vi "continuousSamplingFPGA.vi"() -> ()   [LabVIEW 2012]
uses:
  <vilib>/rvi/Emulation/niFpgaSctlEmulationGetInTimedLoop.vi
  <vilib>/rvi/Emulation/niFpgaSctlEmulationGlobalWrite.vi
  <vilib>/rvi/interface/RandomDataEmulation/nirviRandomDataFPGAFIFO.vi
  <vilib>/rvi/interface/RandomDataEmulation/niFpgaRandomDataHandleErrors.vi
  <vilib>/rvi/eio/common/nirviEmuTemplateMethod_errors.vi
  <vilib>/rvi/DataTransferAndStorage/Container/XNode/niFpgaContainer.xnode
  <vilib>/rvi/interface/RandomDataEmulation/nirviRandomDataFpgaReadWriteTemplate.vi
  <vilib>/eio/EIONode/EIONode.xnode
panel:
  out "z target":bool
  in  "deflection threshold":fxp<+/-,64,32>
  in  "z threshold":fxp<+/-,64,32>
  out "xy target":bool
  in  "y threshold":fxp<+,32,17>
  in  "x threshold":fxp<+,32,17>
  out "z sensor":fxp<+/-,20,5>
  in  "z control":T1
  in  "dataRefresh Clock (uSec)":fxp<+/-,64,29>
  out "Timed Out?":bool
  out "direction":u16
  in  "XY Clock (uSec)":fxp<+/-,64,29>
  out "y sensor":fxp<+/-,20,5>
  out "y output":fxp<+/-,64,29>
  in  "y control":T1
  out "x sensor":fxp<+/-,20,5>
  out "x output":fxp<+/-,64,29>
  in  "x control":T1
  out "deflection sensor":fxp<+/-,20,5>
  out "z output":fxp<+/-,64,29>
  in  "deflection control":T1
  in  "Z Clock (uSec)":fxp<+/-,64,29>
  out "length":u16
  out "y_pos":u16
  out "x_pos":u16
  out "ToRead":u32
  out "signalToStop":bool
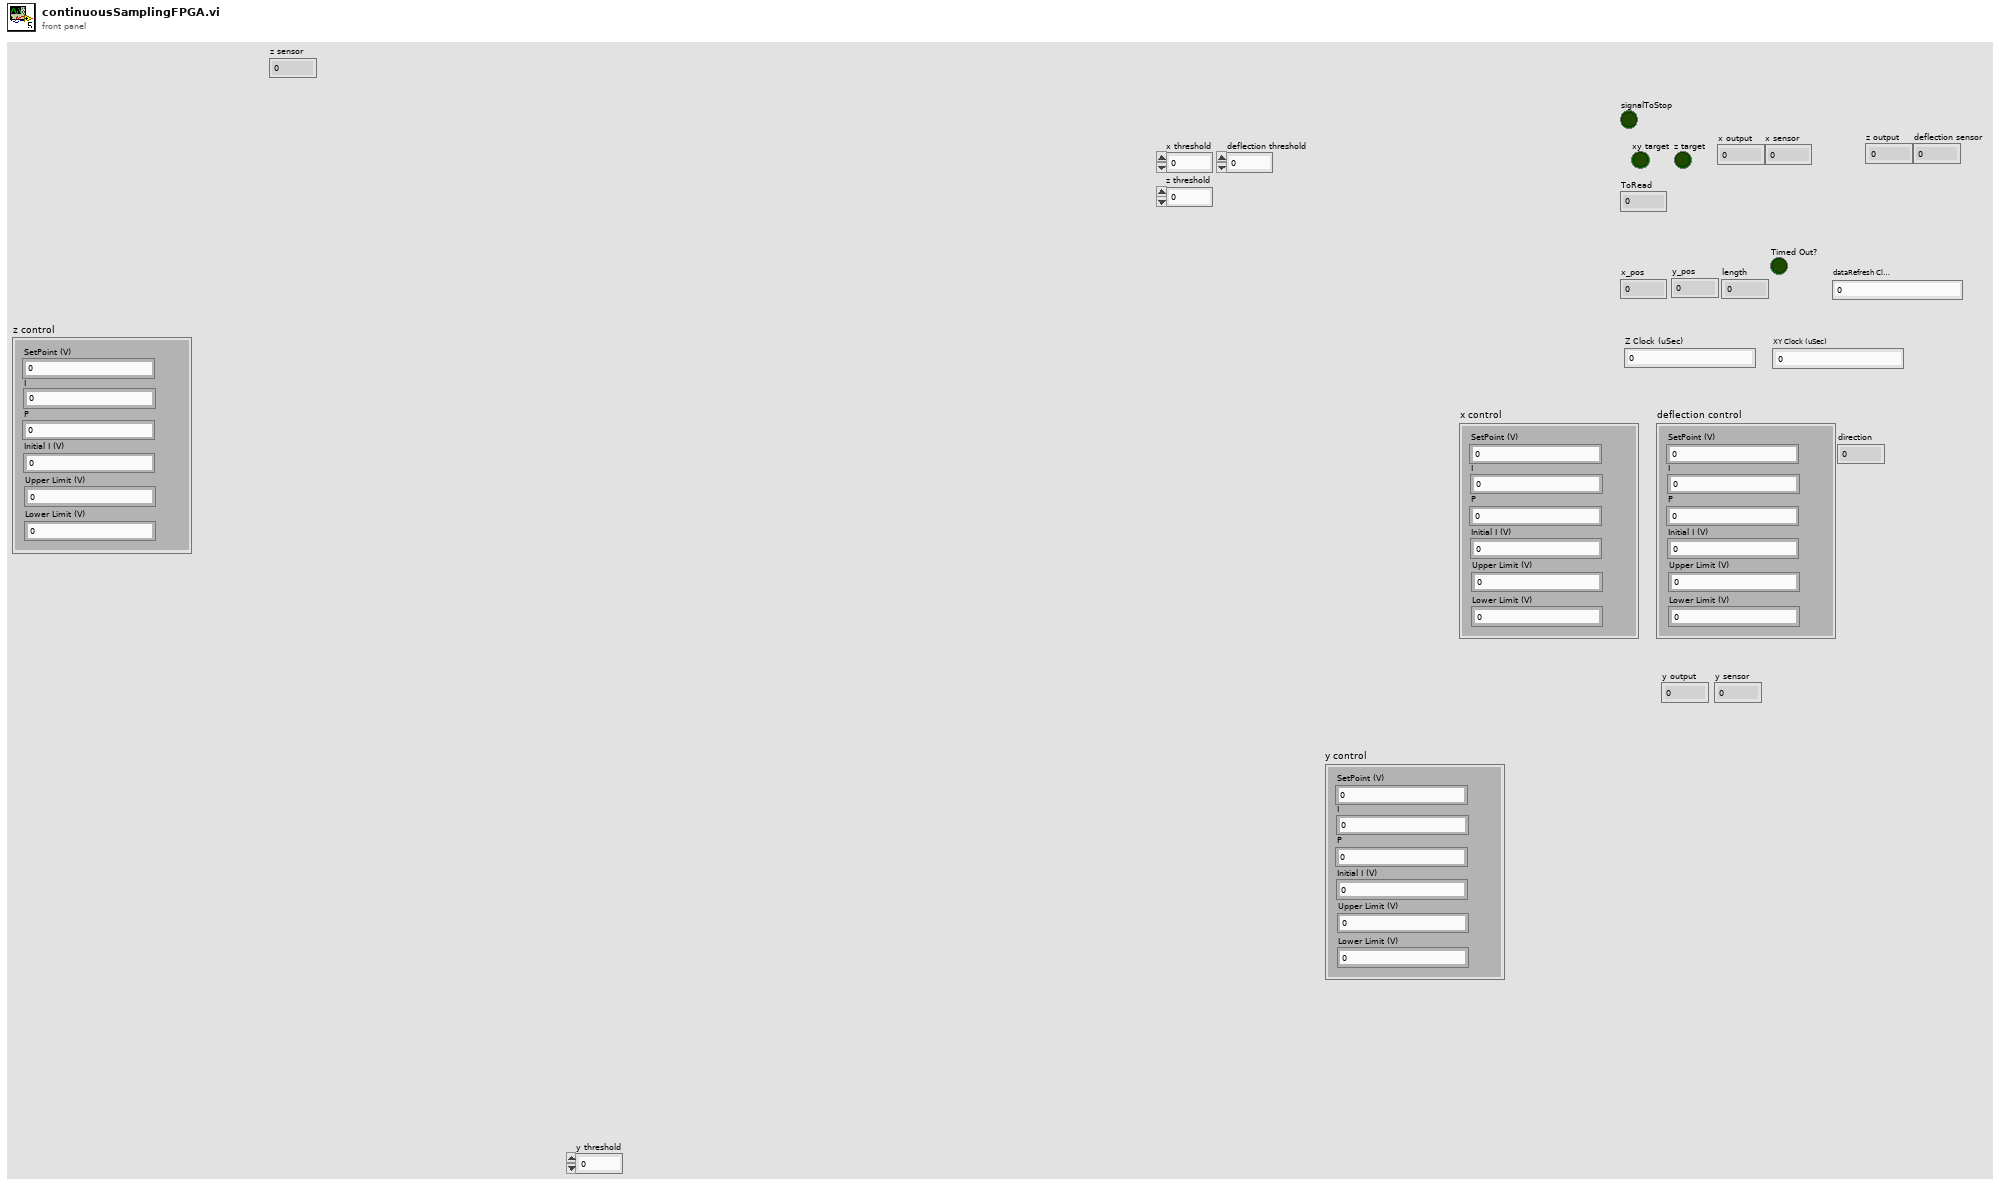
[diagram p1: front panel]
types:
  T1 = cluster{"SetPoint (V)":fxp<+/-,20,5>, "I":fxp<+/-,20,5>, "P":fxp<+/-,20,5>, "Initial I (V)":fxp<+/-,64,29>, "Upper Limit (V)":fxp<+/-,64,29>, "Lower Limit (V)":fxp<+/-,64,29>}
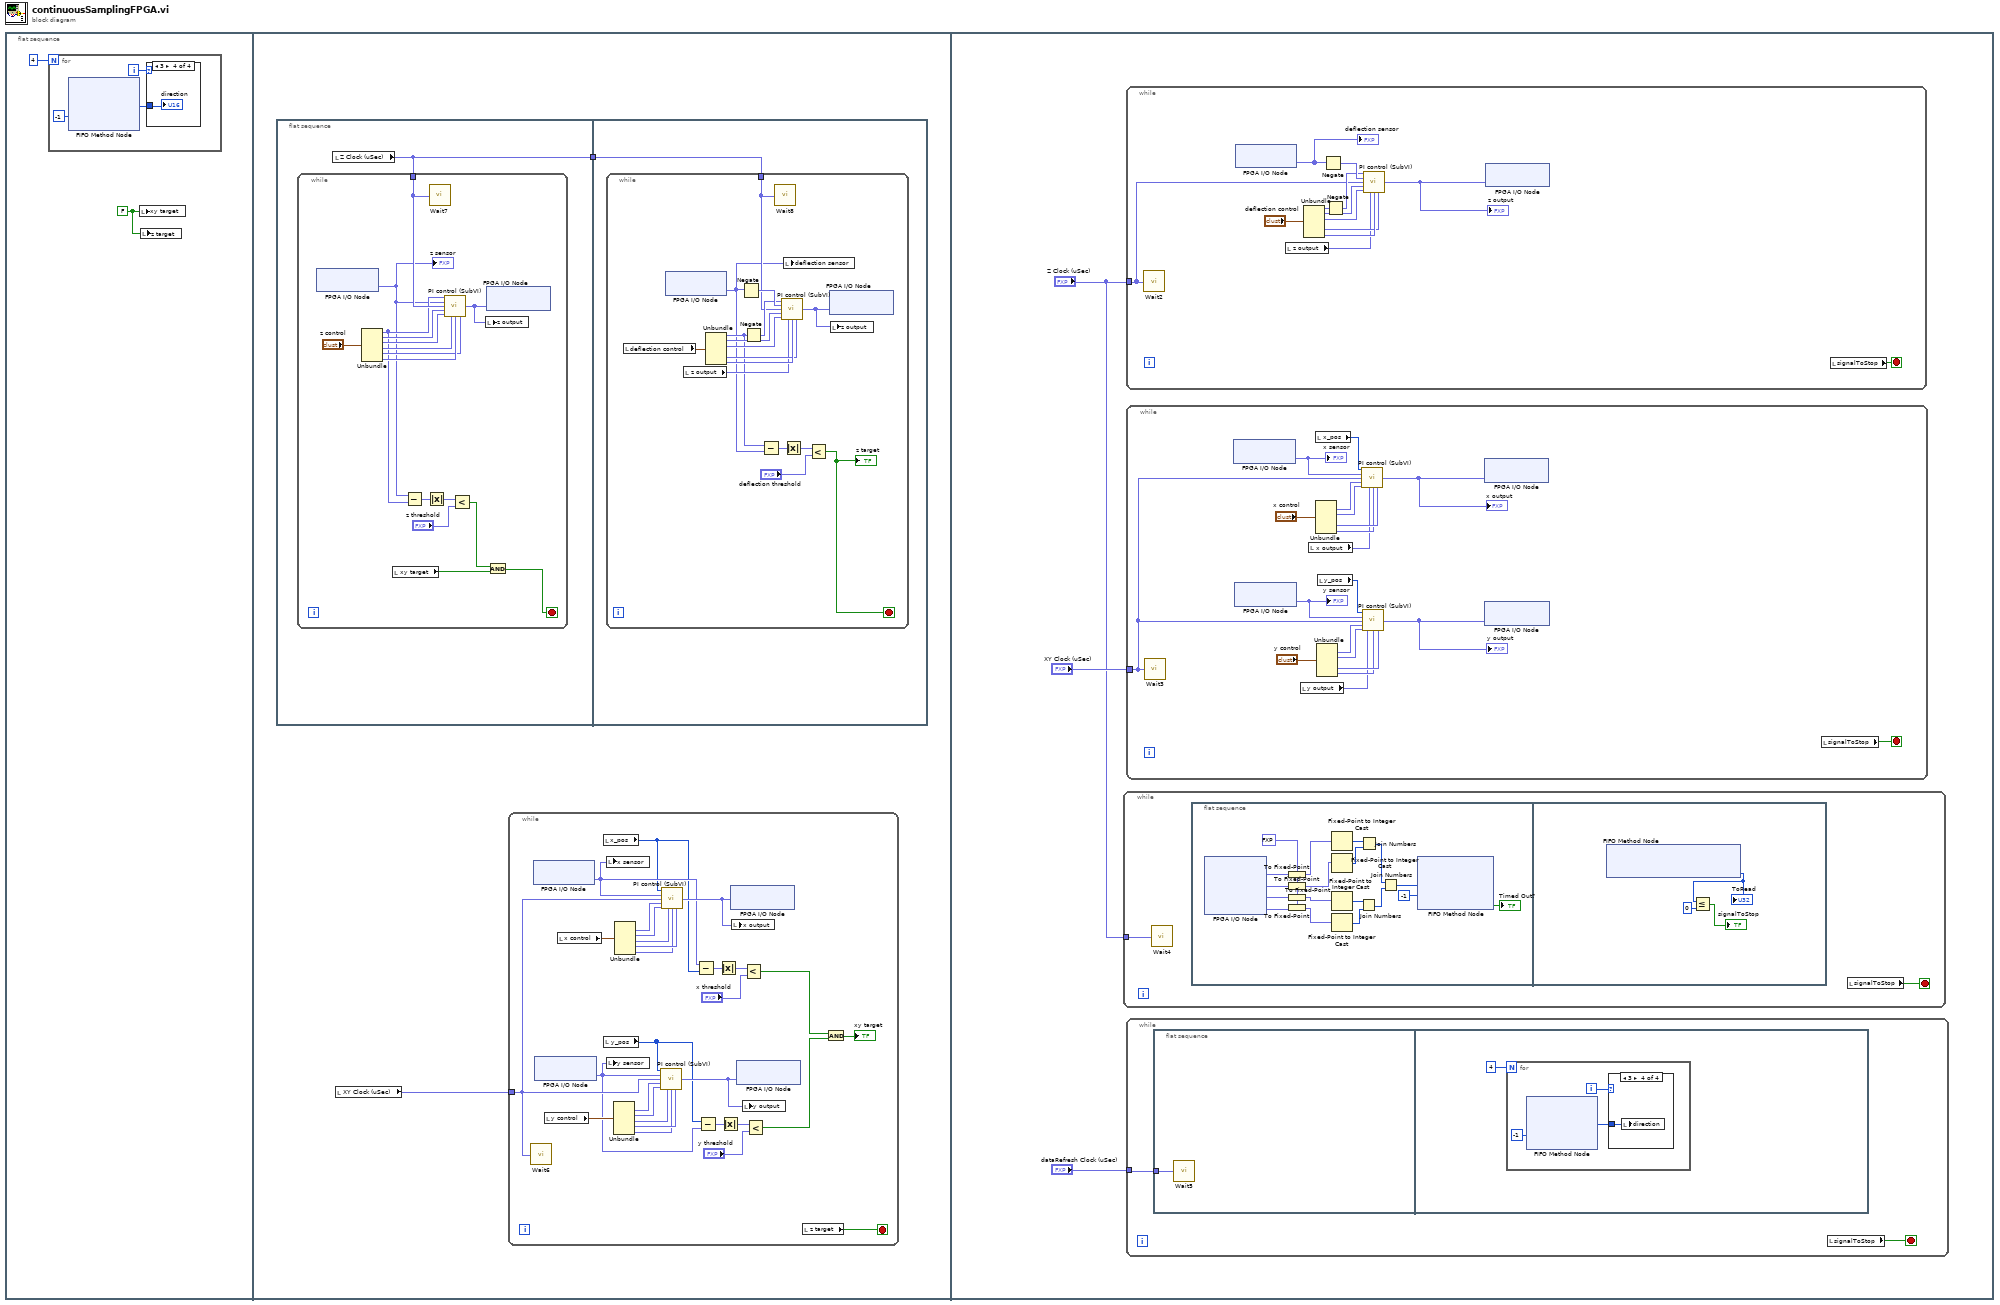
[diagram p0: block diagram]
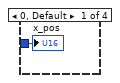
[diagram p2: hidden frame]
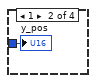
[diagram p3: hidden frame]
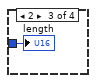
[diagram p4: hidden frame]
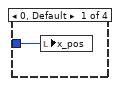
[diagram p5: hidden frame]
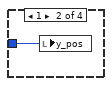
[diagram p6: hidden frame]
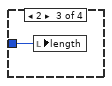
[diagram p7: hidden frame]
diagram:
  n1 = flat-sequence {
    frame #0 {
      w1 = FALSE ("xy target")
      n2 = for {
        N: 4 -> [_]
        i -> [w5]
        n3 = xnode ("FIFO Method Node")("Timeout"=-1) -> ("Element"=w3:u16)  [unwired: 1 in, 2 out]
        n4 = case shown="3" w5 {
          tunnel: w3 -> [w6 w7 w8 w9]
          frame 0, Default {
            "x_pos" <- w6
          }
          frame 1 {
            "y_pos" <- w7
          }
          frame 2 {
            "length" <- w8
          }
          frame 3 {
            "direction" <- w9
          }
        }
      }
      n5 = local write "xy target"(w1) -> ()
      n6 = local write "z target"(w1) -> ()
    }
    frame #1 {
      n7 = flat-sequence {
        tunnel: [w12] -> w10
        tunnel: w10 -> [w29]
        frame #0 {
          n8 = local read "Z Clock (uSec)"() -> (w12:fxp<+/-,64,29>)
          n9 = while {
            tunnel: w12 -> [w21]
            stop <- w19 stop-if-true
            n10 = xnode "FPGA I/O Node"() -> ("Mod1/AI2"=w14:fxp<+/-,20,5>)  [unwired: 1 in, 1 out]
            "z sensor" <- w14
            n11 = Unbundle("z control") -> ("SetPoint (V)"=w15:fxp<+/-,20,5>, "I"=w28:fxp<+/-,20,5>, "P"=w27:fxp<+/-,20,5>, "Initial I (V)"=w26:fxp<+/-,64,29>, "Upper Limit (V)"=w24:fxp<+/-,64,29>, "Lower Limit (V)"=w25:fxp<+/-,64,29>)
            n12 = local read "xy target"() -> (w20:bool)
            n13 = Subtract(x=w14, y=w15) -> (x-y=w18:fxp<+/-,21,6>)
            n14 = Absolute Value(x=w18) -> (abs(x)=w17:fxp<+,20,5>)
            n15 = call "Wait7"("Count(uSec)"=w21) -> ()  [unwired: 1 out]
            n16 = call "PI control (SubVI).vi"("SetPoint"=w15, "Feedback"=w14, "Clock"=w21, "I"=w28, "P"=w27, "Initial I"=w26, "Lower Limit"=w25, "Upper Limit in"=w24) -> ("Output"=w22:fxp<+/-,64,29>)  [unwired: 7 in]
            n17 = Less?(x=w17, y="z threshold") -> (x < y?=w13:bool)
            n18 = local write "z output"(w22) -> ()
            n19 = xnode "FPGA I/O Node"("Mod8/AO2"=w22) -> ()  [unwired: 1 in, 1 out]
            n20 = And(x=w13, y=w20) -> (x .and. y?=w19:bool)
          }
        }
        frame #1 {
          n21 = while {
            tunnel: w29 -> [w37]
            stop <- w30 stop-if-true
            n22 = local read "deflection control"() -> (w38:T1)
            n23 = xnode "FPGA I/O Node"() -> ("Mod1/AI3"=w31:fxp<+/-,20,5>)  [unwired: 1 in, 1 out]
            n24 = local read "z output"() -> (w36:fxp<+/-,64,29>)
            n25 = Unbundle(w38) -> ("SetPoint (V)"=w32:fxp<+/-,20,5>, "I"=w45:fxp<+/-,20,5>, "P"=w44:fxp<+/-,20,5>, "Upper Limit (V)"=w42:fxp<+/-,64,29>, "Lower Limit (V)"=w43:fxp<+/-,64,29>)  [unwired: 1 out]
            n26 = Negate(x=w31) -> (-x=w41:fxp<+/-,21,6>)
            n27 = Negate(x=w32) -> (-x=w40:fxp<+/-,21,6>)
            n28 = Subtract(x=w32, y=w31) -> (x-y=w35:fxp<+/-,21,6>)
            n29 = call "Wait8"("Count(uSec)"=w37) -> ()  [unwired: 1 out]
            n30 = call "PI control (SubVI).vi"("SetPoint"=w40, "Feedback"=w41, "Clock"=w37, "I"=w45, "P"=w44, "Initial I"=w36, "Lower Limit"=w43, "Upper Limit in"=w42) -> ("Output"=w39:fxp<+/-,64,29>)  [unwired: 7 in]
            n31 = Absolute Value(x=w35) -> (abs(x)=w34:fxp<+,20,5>)
            n32 = local write "deflection sensor"(w31) -> ()
            n33 = Less?(x=w34, y="deflection threshold") -> (x < y?=w30:bool)
            "z target" <- w30
            n34 = xnode "FPGA I/O Node"("Mod8/AO2"=w39) -> ()  [unwired: 1 in, 1 out]
            n35 = local write "z output"(w39) -> ()
          }
        }
      }
      n36 = local read "XY Clock (uSec)"() -> (w11:fxp<+/-,64,29>)
      n37 = while {
        tunnel: w11 -> [w61]
        stop <- w46 stop-if-true
        n38 = call "Wait6"("Count(uSec)"=w61) -> ()  [unwired: 1 out]
        n39 = xnode "FPGA I/O Node"() -> ("Mod1/AI0"=w57:fxp<+/-,20,5>)  [unwired: 1 in, 1 out]
        n40 = xnode "FPGA I/O Node"() -> ("Mod1/AI1"=w51:fxp<+/-,20,5>)  [unwired: 1 in, 1 out]
        n41 = local read "y control"() -> (w62:T1)
        n42 = local read "x control"() -> (w69:T1)
        n43 = local read "x_pos"() -> (w56:u16)
        n44 = local read "y_pos"() -> (w50:u16)
        n45 = local write "x sensor"(w57) -> ()
        n46 = local write "y sensor"(w51) -> ()
        n47 = Unbundle(w62) -> ("I"=w63:fxp<+/-,20,5>, "P"=w64:fxp<+/-,20,5>, "Initial I (V)"=w65:fxp<+/-,64,29>, "Upper Limit (V)"=w67:fxp<+/-,64,29>, "Lower Limit (V)"=w66:fxp<+/-,64,29>)  [unwired: 1 out]
        n48 = Unbundle(w69) -> ("I"=w70:fxp<+/-,20,5>, "P"=w71:fxp<+/-,20,5>, "Initial I (V)"=w72:fxp<+/-,64,29>, "Upper Limit (V)"=w74:fxp<+/-,64,29>, "Lower Limit (V)"=w73:fxp<+/-,64,29>)  [unwired: 1 out]
        n49 = call "PI control (SubVI).vi"("SetPoint"=w50, "Feedback"=w51, "Clock"=w61, "I"=w63, "P"=w64, "Initial I"=w65, "Lower Limit"=w66, "Upper Limit in"=w67) -> ("Output"=w60:fxp<+/-,64,29>)  [unwired: 7 in]
        n50 = call "PI control (SubVI).vi"("SetPoint"=w56, "Feedback"=w57, "Clock"=w61, "I"=w70, "P"=w71, "Initial I"=w72, "Lower Limit"=w73, "Upper Limit in"=w74) -> ("Output"=w68:fxp<+/-,64,29>)  [unwired: 7 in]
        n51 = Subtract(x=w57, y=w56) -> (x-y=w59:fxp<+/-,33,18>)
        n52 = Subtract(x=w50, y=w51) -> (x-y=w54:fxp<+/-,33,18>)
        n53 = Absolute Value(x=w59) -> (abs(x)=w58:fxp<+,32,17>)
        n54 = Absolute Value(x=w54) -> (abs(x)=w53:fxp<+,32,17>)
        n55 = xnode "FPGA I/O Node"("Mod8/AO0"=w68) -> ()  [unwired: 1 in, 1 out]
        n56 = local write "x output"(w68) -> ()
        n57 = xnode "FPGA I/O Node"("Mod8/AO1"=w60) -> ()  [unwired: 1 in, 1 out]
        n58 = local write "y output"(w60) -> ()
        n59 = Less?(x=w58, y="x threshold") -> (x < y?=w49:bool)
        n60 = Less?(x=w53, y="y threshold") -> (x < y?=w48:bool)
        n61 = local read "z target"() -> (w46:bool)
        n62 = And(x=w49, y=w48) -> (x .and. y?=→"xy target":bool)
      }
    }
    frame #2 {
      n63 = while {
        tunnel: "Z Clock (uSec)" -> [w90]
        stop <- w89 stop-if-true
        n64 = call "Wait4"("Count(uSec)"=w90) -> ()  [unwired: 1 out]
        n65 = flat-sequence {
          frame #0 {
            w102 = fxp<+/-,32,16> 0.0 ("fixed-point type")
            n66 = xnode "FPGA I/O Node"() -> ("Mod1/AI0"=w106:fxp<+/-,20,5>, "Mod1/AI1"=w103:fxp<+/-,20,5>, "Mod1/AI2"=w104:fxp<+/-,20,5>, "Mod1/AI3"=w105:fxp<+/-,20,5>)  [unwired: 4 in, 4 out]
            n67 = To Fixed-Point(fixed-point type=w102, number=w106) -> (fixed-point=w101:fxp<+/-,32,16>)
            n68 = To Fixed-Point(fixed-point type=w102, number=w103) -> (fixed-point=w100:fxp<+/-,32,16>)
            n69 = To Fixed-Point(fixed-point type=w102, number=w104) -> (fixed-point=w99:fxp<+/-,32,16>)
            n70 = To Fixed-Point(fixed-point type=w102, number=w105) -> (fixed-point=w98:fxp<+/-,32,16>)
            n71 = Fixed-Point to Integer Cast(1:w98) -> (0:w94:i32)
            n72 = Fixed-Point to Integer Cast(1:w101) -> (0:w97:i32)
            n73 = Fixed-Point to Integer Cast(1:w100) -> (0:w96:i32)
            n74 = Fixed-Point to Integer Cast(1:w99) -> (0:w95:i32)
            n75 = Join Numbers(hi=w95, lo=w94) -> ((hi.lo)=w91:u64)
            n76 = Join Numbers(hi=w97, lo=w96) -> ((hi.lo)=w92:u64)
            n77 = Join Numbers(hi=w92, lo=w91) -> ((hi.lo)=w93:u64)
            n78 = xnode ("FIFO Method Node")("Element"=w93, "Timeout"=-1) -> ("Timed Out?"=→"Timed Out?":bool)  [unwired: 1 in, 1 out]
          }
          frame #1 {
            n79 = xnode ("FIFO Method Node")() -> ("Number of Elements to Read"=w111:u32)  [unwired: 1 in, 1 out]
            "ToRead" <- w111
            n80 = Less Or Equal?(x=w111, y=u32 0) -> (x <= y?=→"signalToStop":bool)
          }
        }
        n81 = local read "signalToStop"() -> (w89:bool)
      }
      n82 = while {
        tunnel: "Z Clock (uSec)" -> [w134]
        stop <- w133 stop-if-true
        n83 = call "Wait2"("Count(uSec)"=w134) -> ()  [unwired: 1 out]
        n84 = xnode "FPGA I/O Node"() -> ("Mod1/AI3"=w138:fxp<+/-,20,5>)  [unwired: 1 in, 1 out]
        "deflection sensor" <- w138
        n85 = local read "z output"() -> (w132:fxp<+/-,64,29>)
        n86 = Unbundle("deflection control") -> ("SetPoint (V)"=w136:fxp<+/-,20,5>, "I"=w144:fxp<+/-,20,5>, "P"=w143:fxp<+/-,20,5>, "Upper Limit (V)"=w141:fxp<+/-,64,29>, "Lower Limit (V)"=w142:fxp<+/-,64,29>)  [unwired: 1 out]
        n87 = Negate(x=w138) -> (-x=w137:fxp<+/-,21,6>)
        n88 = Negate(x=w136) -> (-x=w135:fxp<+/-,21,6>)
        n89 = call "PI control (SubVI).vi"("SetPoint"=w135, "Feedback"=w137, "Clock"=w134, "I"=w144, "P"=w143, "Initial I"=w132, "Lower Limit"=w142, "Upper Limit in"=w141) -> ("Output"=w140:fxp<+/-,64,29>)  [unwired: 7 in]
        "z output" <- w140
        n90 = xnode "FPGA I/O Node"("Mod8/AO2"=w140) -> ()  [unwired: 1 in, 1 out]
        n91 = local read "signalToStop"() -> (w133:bool)
      }
      n92 = while {
        tunnel: "dataRefresh Clock (uSec)" -> [w79]
        stop <- w78 stop-if-true
        n93 = flat-sequence {
          tunnel: w79 -> [w80]
          frame #0 {
            n94 = call "Wait5"("Count(uSec)"=w80) -> ()  [unwired: 1 out]
          }
          frame #1 {
            n95 = for {
              N: 4 -> [_]
              i -> [w84]
              n96 = xnode ("FIFO Method Node")("Timeout"=-1) -> ("Element"=w82:u16)  [unwired: 1 in, 2 out]
              n97 = case shown="3" w84 {
                tunnel: w82 -> [w85 w86 w87 w88]
                frame 0, Default {
                  n98 = local write "x_pos"(w85) -> ()
                }
                frame 1 {
                  n99 = local write "y_pos"(w86) -> ()
                }
                frame 2 {
                  n100 = local write "length"(w87) -> ()
                }
                frame 3 {
                  n101 = local write "direction"(w88) -> ()
                }
              }
            }
          }
        }
        n102 = local read "signalToStop"() -> (w78:bool)
      }
      n103 = while {
        tunnel: "XY Clock (uSec)" -> [w117]
        stop <- w114 stop-if-true
        n104 = call "Wait3"("Count(uSec)"=w117) -> ()  [unwired: 1 out]
        n105 = xnode "FPGA I/O Node"() -> ("Mod1/AI0"=w124:fxp<+/-,20,5>)  [unwired: 1 in, 1 out]
        "x sensor" <- w124
        n106 = xnode "FPGA I/O Node"() -> ("Mod1/AI1"=w131:fxp<+/-,20,5>)  [unwired: 1 in, 1 out]
        "y sensor" <- w131
        n107 = local read "y output"() -> (w112:fxp<+/-,64,29>)
        n108 = local read "x output"() -> (w113:fxp<+/-,64,29>)
        n109 = Unbundle("x control") -> ("I"=w118:fxp<+/-,20,5>, "P"=w119:fxp<+/-,20,5>, "Upper Limit (V)"=w121:fxp<+/-,64,29>, "Lower Limit (V)"=w120:fxp<+/-,64,29>)  [unwired: 2 out]
        n110 = local read "x_pos"() -> (w115:u16)
        n111 = Unbundle("y control") -> ("I"=w125:fxp<+/-,20,5>, "P"=w126:fxp<+/-,20,5>, "Upper Limit (V)"=w128:fxp<+/-,64,29>, "Lower Limit (V)"=w127:fxp<+/-,64,29>)  [unwired: 2 out]
        n112 = local read "y_pos"() -> (w116:u16)
        n113 = call "PI control (SubVI).vi"("SetPoint"=w115, "Feedback"=w124, "Clock"=w117, "I"=w118, "P"=w119, "Initial I"=w113, "Lower Limit"=w120, "Upper Limit in"=w121) -> ("Output"=w122:fxp<+/-,64,29>)  [unwired: 7 in]
        "x output" <- w122
        n114 = call "PI control (SubVI).vi"("SetPoint"=w116, "Feedback"=w131, "Clock"=w117, "I"=w125, "P"=w126, "Initial I"=w112, "Lower Limit"=w127, "Upper Limit in"=w128) -> ("Output"=w129:fxp<+/-,64,29>)  [unwired: 7 in]
        "y output" <- w129
        n115 = xnode "FPGA I/O Node"("Mod8/AO0"=w122) -> ()  [unwired: 1 in, 1 out]
        n116 = xnode "FPGA I/O Node"("Mod8/AO1"=w129) -> ()  [unwired: 1 in, 1 out]
        n117 = local read "signalToStop"() -> (w114:bool)
      }
    }
  }
